vi "SetGreenLevel.vi"(2 "error in":errorcluster, 3 "Green Light Level":sgl) -> (0 "error out":errorcluster)   [LabVIEW 2012]
uses:
  <userlib>/ROSforLV/ROS/Code/Console/Servers/ServerSubs/TopicDef.ctl
  <userlib>/ROSforLV/ROS/Code/SubVIs/_ROSDirection.ctl
  <userlib>/ROSforLV/ROS/MessageBuilding/std_msgs/subs/float32Scalar.vi
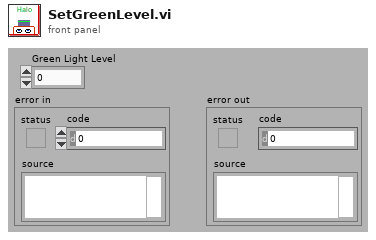
[diagram p1: front panel]
types:
  T1 = typedef "TopicDef.ctl" = cluster{"Topic":string, "Type":string, "Action":T2, "Update (ms)":u16, "write queue":u16}
  T2 = typedef "_ROSDirection.ctl" = enum16{"Node", "Publisher", "Subscriber", "Service Client"}
  T3 = typedef "_ROSControl.ctl" = cluster{"topic port":u16, "Node":string, "topic":string, "type":string, "node port":u16, "error ":errorcluster, "Direction":T2, "APIs":string[], "Update (ms)":u16, "write queue":u16}
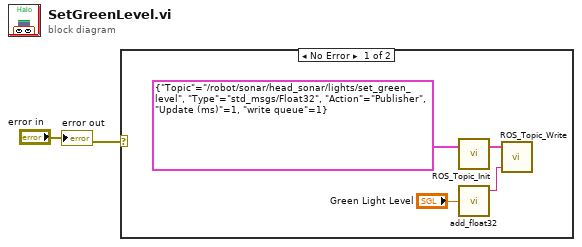
[diagram p0: block diagram]
diagram:
  n1 = case shown="No Error" "error in" {
    frame No Error {
      n2 = call <userlib>:"ROS_Topic_Init.vi"("Definitions"=T1 {"Topic"="/robot/sonar/head_sonar/lights/set_green_level", "Type"="std_msgs/Float32", "Action"=enum."Publisher", "Update (ms)"=1, "write queue"=1}) -> ("ROS out"=w5:T3)  [unwired: 2 in]
      n3 = call-poly <userlib>:"add_float32.vi"("Numeric"="Green Light Level") -> ("msg out"=w4:string)  [unwired: 4 in]
      n4 = call <userlib>:"ROS_Topic_Write.vi"("Msg in"=w4, "ROS in"=w5) -> ()  [unwired: 2 in, 1 out]
    }
    frame Error {
    }
  }
  "error out" <- "error in"
